vi "Reinitalize Components.vi"(8 "error in (no error)":errorcluster, 11 "Panel in":refnum<class "Panel.lvclass">) -> (0 "error out":errorcluster, 3 "Panel out":refnum<class "Panel.lvclass">)   [LabVIEW 2021, in "Panel.lvlib" / "Panel.lvclass"]
uses:
  Panel.lvclass
  Panel.lvclass/Panel.ctl
  Type Defs/Tester Rx Dataset.ctl
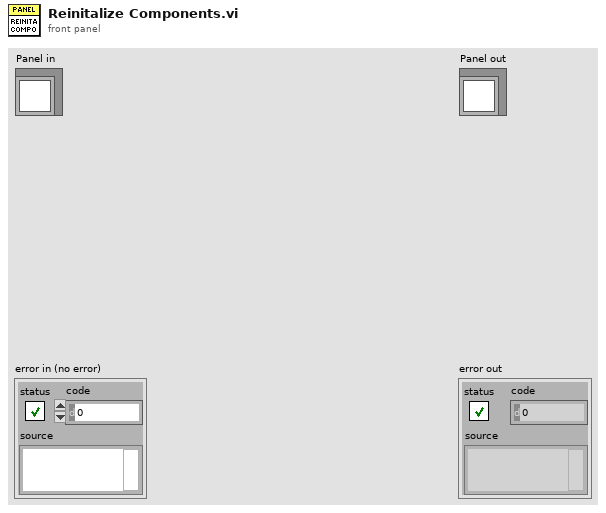
[diagram p1: front panel]
types:
  T1 = typedef "Panel.lvlib/Panel.lvclass/Tester Rx Dataset.ctl" = cluster{"Start":bool, "NestStatus":bool, "PalletID":u32, "BarcodeData":string, "StepEcho":u32, "Cylinder_1":bool, "Cylinder_2":bool, "Cylinder_3":bool, "Cylinder_4":bool, "Cylinder_5":bool, "ResultsAck":bool, "Reset":bool, "Stop":bool, "FaultCode":u32}
  T2 = typedef "Panel.lvlib/Panel.lvclass/Tester Tx Dataset.ctl" = cluster{"Fault":bool, "StepNo":u32, "Ready":bool, "HighVoltage":bool, "TestRunning":bool, "ResultsReady":bool, "Results":u32, "ElapsedTime":u32, "Online":bool, "TimeCompleted":i32[], "Timeout":bool}
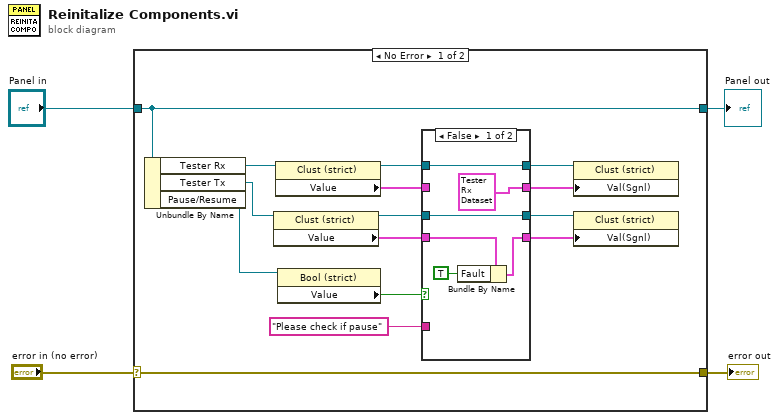
[diagram p0: block diagram]
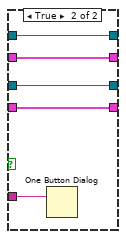
[diagram p2: hidden frame]
diagram:
  n1 = case shown="No Error" "error in (no error)" {
    selector: "error in (no error)" -> [w19 w32]
    tunnel: [w19 w32] -> w3
    tunnel: [w18 w31] -> w1
    tunnel: "Panel in" -> [w18 w31]
    frame No Error {
      n2 = Unbundle By Name(w18) -> ("Tester Rx"=w17:refnum<vi>, "Tester Tx"=w11:refnum<vi>, "Pause/Resume"=w16:refnum<vi>)
      n3 = property class="Clust (strict)"(reference=w11) -> (reference out=w8:refnum<vi>, "Value"=w6:T2)  [unwired: 1 in, 1 out]
      n4 = property class="Clust (strict)"(reference=w17) -> (reference out=w10:refnum<vi>, "Value"=w13:T1)  [unwired: 1 in, 1 out]
      n5 = property class="Bool (strict)"(reference=w16) -> ("Value"=w15:bool)  [unwired: 1 in, 2 out]
      n6 = case shown="False" w15 {
        tunnel: [T1 {"Start"=FALSE, "NestStatus"=FALSE, "PalletID"=0, "BarcodeData"="P:10-000001R:04S:QMC2200001", "StepEcho"=0, "Cylinder_1"=FALSE, "Cylinder_2"=FALSE, "Cylinder_3"=FALSE, "Cylinder_4"=FALSE, "Cylinder_5"=FALSE, "ResultsAck"=FALSE, "Reset"=FALSE, "Stop"=FALSE, "FaultCode"=0} ("Value") w30] -> w14
        tunnel: w13 -> [_ w30]
        tunnel: "Please check if pause" ("message") -> [_ w29]
        tunnel: w10 -> [w24 w28]
        tunnel: [w24 w28] -> w9
        tunnel: w8 -> [w23 w27]
        tunnel: [w23 w27] -> w7
        tunnel: w6 -> [w22 w26]
        tunnel: [w20 w26] -> w5
        frame False {
          n7 = Bundle By Name(cluster=w22, "Fault"=TRUE) -> (w20:T2)
        }
        frame True {
          n8 = One Button Dialog(message=w29) -> ()  [unwired: 1 in, 1 out]
        }
      }
      n9 = property class="Clust (strict)"(reference=w9, "Val(Sgnl)"=w14) -> ()  [unwired: 1 in, 2 out]
      n10 = property class="Clust (strict)"(reference=w7, "Val(Sgnl)"=w5) -> ()  [unwired: 1 in, 2 out]
    }
    frame Error {
    }
  }
  "error out" <- w3
  "Panel out" <- w1
